vi "Global config keb.vi"() -> ()   [LabVIEW 2019]
uses:
  ConfigurazioneKeb.ctl
panel:
  in  "Tensione Target KEB":dbl
  in  "Configurazione keb":T1
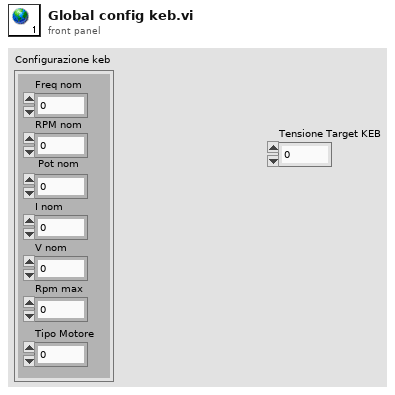
[diagram p1: front panel]
types:
  T1 = typedef "ConfigurazioneKeb.ctl" = cluster{"Freq nom":dbl, "RPM nom":dbl, "Pot nom":dbl, "I nom":dbl, "V nom":dbl, "Rpm max":dbl, "Tipo Motore":dbl}
diagram:
